vi "Raise Error (no overwrite).vi"(8 "error in":errorcluster, 11 "Error Message":string) -> (0 "error out":errorcluster)   [LabVIEW 2020]
doc: "Raises a custom, user-generated error if and only if there is no error at the \"error in\" input.\n\nIn other words, this VI does not overwrite an existing error. This behaviour is believed to be desirable in most cases."
panel:
  # "Development\ncontrols/indicators useful for development and testing, but which are not outputs of the VI"
  # "Input\nInputs to the VI"
  # "Output\nOutputs of the VI"
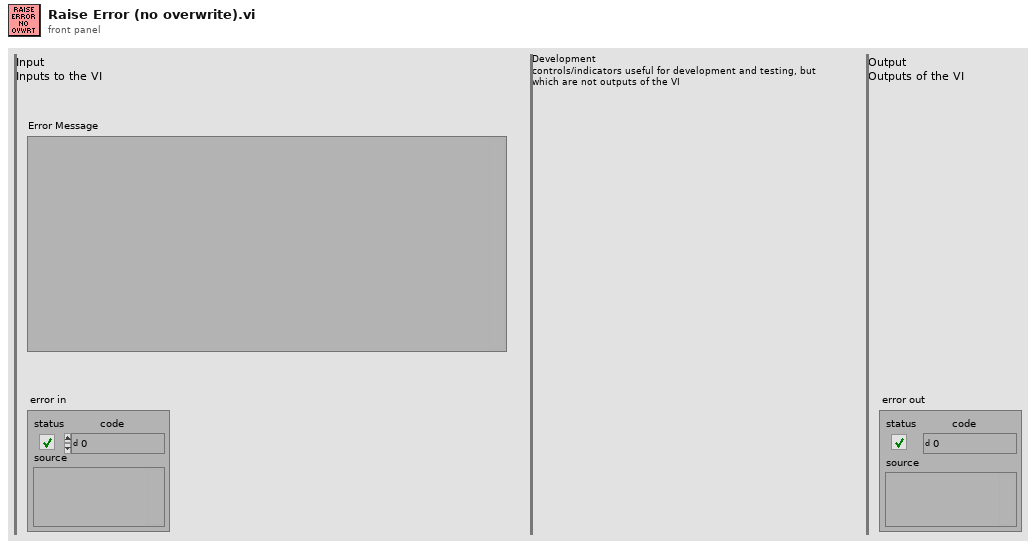
[diagram p1: front panel]
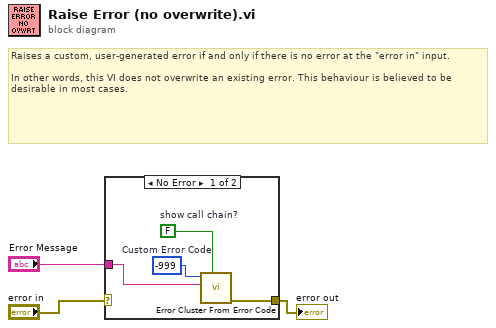
[diagram p0: block diagram]
diagram:
  # "Raises a custom, user-generated error if and only if there is no error at the \"error in\" input.\n\nIn other words, this VI does not overwrite an existing error. This behaviour is believed to be desirable in most cases."
  n1 = case shown="No Error" "error in" {
    selector: "error in" -> [_ w8]
    tunnel: [w7 w8] -> w2
    tunnel: "Error Message" -> [w5 _]
    frame No Error {
      w4 = FALSE  # show call chain?
      w6 = -999  # Custom Error Code
      n2 = call <vilib>:"Error Cluster From Error Code.vi"("show call chain? (False)"=w4, "error message (\"\")"=w5, "error code (0)"=w6) -> ("error out"=w7:errorcluster)  [unwired: 6 in]
    }
    frame Error {
    }
  }
  "error out" <- w2
